vi "写入excel数据.vi"(4 "OUT":i32=4, 5 "IN":i32=128, 6 "testType":string, 7 "ref":bool=TRUE, 8 "error in (no error)":errorcluster, 10 "style":string="dCOM%d", 11 "NI_report in":refnum<class "NI_report.lvclass">) -> (0 "error out":errorcluster, 3 "NI_report out":refnum<class "NI_report.lvclass">)   [LabVIEW 2015]
uses:
  <vilib>/Utility/NIReport.llb/NI_report.lvclass
  <vilib>/addons/_office/excel.llb/Excel Easy Table (str).vi
  <vilib>/Utility/NIReport.llb/Excel/NI_Excel.lvclass
  <vilib>/addons/_office/NI_ReportGenerationToolkit.lvlib
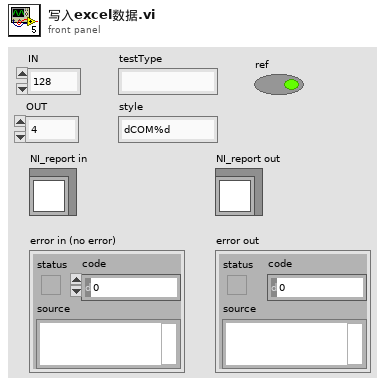
[diagram p1: front panel]
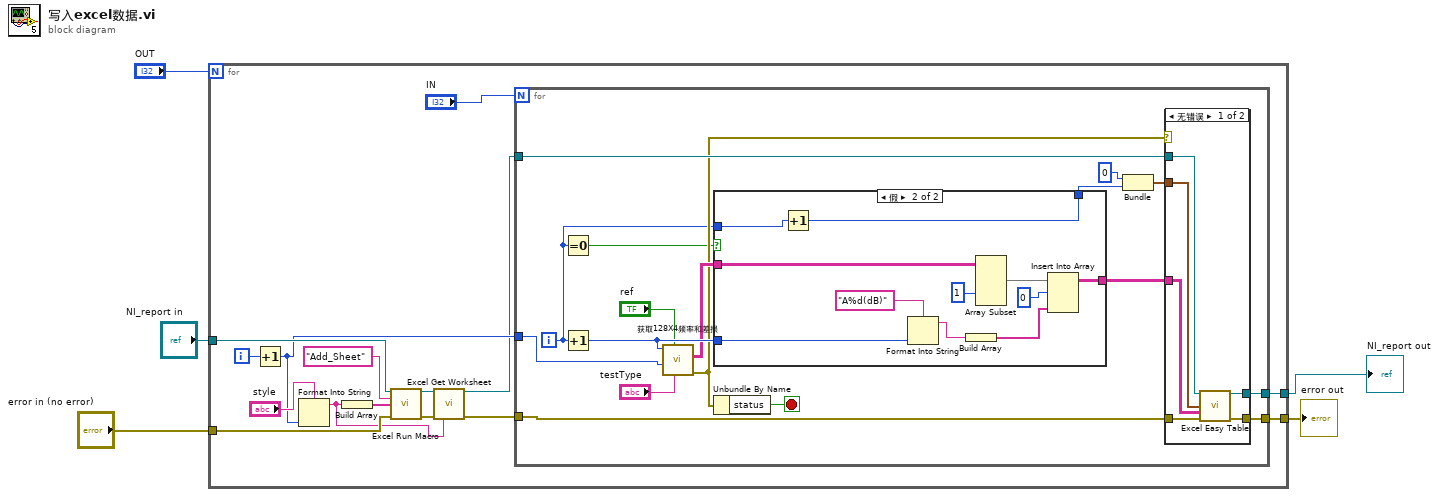
[diagram p0: block diagram]
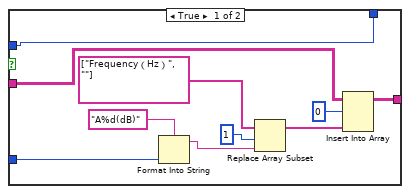
[diagram p2: hidden frame]
diagram:
  n1 = for {
    N: "OUT" -> [_]
    tunnel: "NI_report in" -> [w18]
    tunnel: "error in (no error)" -> [w17]
    tunnel: [w7] -> w4
    tunnel: [w6] -> w5
    i -> [w13]
    n2 = Increment(x=w13) -> (x+1=w10:i32)
    n3 = Format Into String(format string="style", w10) -> (resulting string=w11:string)  [unwired: 2 in, 1 out]
    n4 = Build Array(w11) -> (w15:string[])
    n5 = call <vilib>:"Excel Run Macro.vi"("report in"=w18, "macro name"="Add_Sheet", "parameters"=w15, "error in (no error)"=w17) -> ("report out"=w20:refnum<class "NI_report.lvclass">, "error out"=w16:errorcluster)  [unwired: 9 in, 1 out]
    n6 = call <vilib>:"Excel Get Worksheet.vi"("report in"=w20, "error in (no error)"=w16, "name (\"\")"=w11) -> ("report out"=w9:refnum<class "NI_report.lvclass">, "error out"=w8:errorcluster)  [unwired: 11 in]
    n7 = for {
      N: "IN" -> [_]
      tunnel: w10 -> [w37]
      tunnel: w9 -> [w34]
      tunnel: w8 -> [w33]
      tunnel: [w27] -> w7
      tunnel: [w26] -> w6
      i -> [w21]
      stop <- w29 stop-if-true
      n8 = Equal To 0?(x=w21) -> (x = 0?=w24:bool)
      n9 = Increment(x=w21) -> (x+1=w36:i32)
      n10 = call "获取128X4频率和差损.vi"("testType"="testType", "ref"="ref", "COM"=w37, "A"=w36) -> ("error out"=w28:errorcluster, "Freq&S21"=w35:string[][])  [unwired: 6 in]
      n11 = case shown="假" w24 {
        tunnel: w36 -> [w47 w58]
        tunnel: w35 -> [w42 w54]
        tunnel: [w39 w55] -> w32
        tunnel: [w38 w48] -> w22
        tunnel: w21 -> [w38 w49]
        frame True {
          n12 = Format Into String(format string="A%d(dB)", w47) -> (resulting string=w43:string)  [unwired: 2 in, 1 out]
          n13 = Replace Array Subset(array=string[] ["Frequency（Hz）", ""] ("new element/subarray"), new element=w43, index=1) -> (w40:string[])
          n14 = Insert Into Array(array=w42, index (row)=0, new element=w40) -> (w39:string[][])  [unwired: 1 in]
        }
        frame False {
          n15 = Increment(x=w49) -> (x+1=w48:i32)
          n16 = Format Into String(format string="A%d(dB)", w58) -> (resulting string=w51:string)  [unwired: 2 in, 1 out]
          n17 = Build Array(w51) -> (w50:string[])
          n18 = Array Subset(array=w54, index (col)=1 ("disabled index (col)")) -> (w52:string[][])  [unwired: 3 in]
          n19 = Insert Into Array(array=w52, index (row)=0, new element=w50) -> (w55:string[][])  [unwired: 1 in]
        }
      }
      n20 = Unbundle By Name(w28) -> ("status"=w29:bool)
      n21 = Bundle(0, w22) -> (w30:cluster{i32, i32})  [unwired: 1 in]
      n22 = case shown="无错误" w28 {
        tunnel: w34 -> [w64 w66]
        tunnel: w33 -> [w63 w65]
        tunnel: w32 -> [w62 _]
        tunnel: w30 -> [w61 _]
        tunnel: [w60 w66] -> w27
        tunnel: [w59 w65] -> w26
        frame No Error {
          n23 = call-poly <vilib>:"Excel Easy Table.vi"("report in"=w64, "start (0, 0)"=w61, "text data"=w62, "error in (no error)"=w63) -> ("report out"=w60:refnum<class "NI_report.lvclass">, "error out"=w59:errorcluster)  [unwired: 7 in, 3 out]
        }
        frame Error {
        }
      }
    }
  }
  "error out" <- w5
  "NI_report out" <- w4
